vi "Interpolation Solver_worksheet.vi"(7 "method":T2(ring)=enum."Spline", 9 "factor":i32=11) -> ()   [LabVIEW 2021]
doc: "Demonstrates different types of interpolation on a set of raw data. The types of interpolation demonstrated in this example are Linear, Polynomial, Spline, and Rational."
uses:
  <vilib>/Analysis/NI_AALPro.lvlib
panel:
  out "Interpolated and sampled":string
  in  "Temp sampling":string="-2.2E-4\t4758.78\t1E-4\t2721.471\t-5E-5\t2008\t-5E-5\t1685\t1E-4\t1450\t1E-4\t1164.85\t-0.29989\t764.0274\n0.30011\t4462.235\t0.3\t2648\t0.30005\t1987.353\t0.30005\t1669\t1.1E-4\t1450\t0.29994\t1163\t-1.1E-4\t762.4022\n0.60005\t4148.875\t0.59999\t2535.23\t0.60005\t1930\t0.59994\t1632\t0.29994\t1442\t0.59999\t1154\t5E-5\t758.3495\n0.89999\t3924.31\t0.89999\t2443\t0.89993\t1879\t0.89999\t1596\t0.3\t1442\t0.9001\t1141\t0.29983\t759.8404\n1.19998\t3754.89\t1.19998\t2370\t1.19998\t1836\t1.19998\t1566\t0.59999\t1420\t1.20004\t1129.09\t0.3\t757.0791\n1.49993\t3615.25\t1.49993\t2311.24\t1.49998\t1800.059\t1.49998\t1539.437\t0.60005\t1419.15\t1.49993\t1118\t0.59994\t754.8484\n1.79992\t3502.73\t1.80003\t2261.312\t1.79987\t1771\t1.80003\t1516\t0.89999\t1395\t1.79992\t1108\t0.89999\t751.6615\n2.09992\t3405.49\t2.10003\t2219\t2.09992\t1747.25\t2.10036\t1496\t0.9001\t1395\t2.09992\t1099.24\t1.19998\t748.4732\n2.39997\t3317.85\t2.40008\t2181\t2.40008\t1728.235\t2.39997\t1478\t1.19988\t1373\t2.40002\t1092\t1.50004\t745.1494\n2.70008\t3247\t2.69997\t2147.36\t2.69997\t1712\t2.69991\t1460\t1.20004\t1373.353\t2.69997\t1085\t1.79998\t741.0916\n2.99991\t3177.43\t2.99996\t2122.941\t3.00007\t1699\t2.99996\t1447\t1.49998\t1354.235\t2.99991\t1079\t2.09997\t737.0983\n3.29996\t3122.62\t3.29996\t2096\t3.29996\t1687\t3.29996\t1435\t1.49998\t1354\t3.29996\t1073\t2.39992\t733.8118\n3.59995\t3072\t3.60001\t2074\t3.60001\t1676\t3.5999\t1425\t1.79992\t1338\t3.59995\t1068\t2.70002\t730.3677\n3.89995\t3024\t3.90011\t2054\t3.90001\t1666.537\t3.90006\t1416\t1.79998\t1336\t3.90011\t1063\t3.00007\t728.4455\n4.20006\t2982\t4.2\t2035.625\t4.19995\t1657.937\t4.2\t1406.937\t2.09986\t1319.059\t4.20006\t1059\t3.29996\t725.281\n4.49989\t2940.19\t4.49994\t2018.473\t4.49994\t1650\t4.49994\t1398\t2.09992\t1323\t4.49989\t1054.911\t3.60001\t723.3808\n4.79994\t2898\t4.79988\t2002.706\t4.79994\t1642.062\t4.80005\t1390.437\t2.39997\t1310\t4.79999\t1052\t3.90001\t721.5694\n5.09988\t2857.15\t5.09999\t1988\t5.10004\t1635\t5.09999\t1383.235\t2.40002\t1305\t5.09994\t1048.125\t4.2\t719.9192\n5.39993\t2811.62\t5.39999\t1974.187\t5.39999\t1629\t5.39999\t1377\t2.69997\t1298.57\t5.39999\t1046\t4.50005\t717.7494\n5.69998\t2746.67\t5.69998\t1962\t5.69998\t1622\t5.69993\t1371\t2.70002\t1291\t5.69998\t1043.84\t4.79994\t716.1806\n5.99998\t2712.765\t5.99987\t1950.04\t5.99998\t1616\t6.00009\t1364.789\t2.99996\t1278\t8.09995\t1018\t5.09994\t714.4917\n6.29997\t2692\t6.29987\t1939\t6.30003\t1610\t6.29992\t1359\t3.00002\t1287\t8.39989\t1015.588\t5.39999\t713.1643\n6.59997\t2672\t6.59992\t1928.157\t6.59986\t1604\t6.59992\t1354\t3.2999\t1265.792\t8.7\t1013\t5.70004\t711.2428\n6.89997\t2652.41\t6.90002\t1918\t6.89997\t1598\t6.89991\t1349\t3.30001\t1277.412\t9\t1011.39\t5.99998\t709.8922\n7.19996\t2632.31\t7.20002\t1908\t7.20007\t1592.78\t7.20007\t1344\t3.60001\t1269\t9.59993\t1007\t6.29992\t707.9154\n7.49996\t2613\t7.50001\t1899\t7.49991\t1587.19\t7.50001\t1339\t3.90001\t1260\t9.89998\t1004\t6.59992\t705.745\n7.79996\t2595.12\t7.79996\t1890\t7.79996\t1582\t7.80007\t1335\t4.19995\t1252\t10.19993\t1001\t6.89997\t704.6705\n8.09995\t2579\t8.09995\t1881\t8.10001\t1577\t8.0999\t1330\t4.49994\t1245\t10.49987\t998.8081\t7.19996\t702.9026\n8.39995\t2564\t8.40011\t1872\t8.39989\t1572.25\t8.39995\t1326\t4.79999\t1238\t10.80008\t996.05\t7.50001\t700.9308\n8.69994\t2549.75\t8.69989\t1865\t8.7\t1568\t8.70005\t1321\t5.09994\t1231\t11.09997\t994\t7.80001\t699.1752\n9\t2538\t8.99989\t1858\t9\t1563.882\t9\t1317.5\t5.39999\t1224\t11.39997\t992\t8.09995\t697.7639\n9.29994\t2527\t9.29994\t1852\t9.29994\t1559\t9.29994\t1313.706\t5.69993\t1217.294\t11.69991\t989.5833\t8.39989\t696.1505\n9.60004\t2516\t9.59993\t1845.634\t9.59999\t1555\t9.59993\t1310\t5.99998\t1211\t11.99996\t987.8235\t8.70005\t694.8553\n9.89987\t2508\t9.90004\t1840.48\t9.90004\t1551\t9.90009\t1306\t6.29997\t1205\t12.2999\t985.9565\t9\t692.7788\n10.19987\t2500.832\t10.19987\t1835.812\t10.19993\t1547.081\t10.19998\t1302\t6.60003\t1199.412\t12.59995\t983.7073\t9.29988\t691.7825\n10.50003\t2494.312\t10.49998\t1831\t10.49992\t1543.706\t10.50009\t1298.059\t6.89991\t1194\t12.89995\t981.303\t9.59993\t690.9664\n10.79997\t2489\t10.79992\t1826.059\t10.79986\t1539.824\t10.79997\t1295\t7.19996\t1188.812\t13.19989\t980\t9.90004\t689.5472\n11.10002\t2483\t11.09986\t1796.16\t11.09997\t1536\t11.10008\t1291\t7.50001\t1183\t13.50005\t977.6444\t10.19998\t688.6897\n11.40002\t2480.28\t11.39997\t1794.7\t11.39991\t1532\t11.39991\t1288\t7.7999\t1178\t13.79993\t974.67\t10.49998\t687.2567\n11.70002\t2475.706\t11.69996\t1790.53\t11.70002\t1529\t11.69991\t1284\t8.09995\t1172.294\t14.09999\t972\t10.79992\t686.3817\n11.99996\t2471\t12.00001\t1784.5\t11.9999\t1525\t12.00012\t1280\t8.4\t1167\t14.39998\t970\t11.09997\t684.9439\n12.2999\t2467\t12.29995\t1779.92\t12.29995\t1522\t12.29995\t1277\t8.7\t1161\t14.69998\t968\t11.40002\t683.9548\n12.60006\t2461.21\t12.6\t1775.3\t12.5999\t1518\t12.6\t1273.687\t8.99994\t1156\t14.99997\t965.81\t11.70007\t682.3112\n12.90006\t2456\t12.90006\t1770.63\t12.89995\t1514.86\t12.90006\t1270\t9.29999\t1152.494\t15.29997\t964\t11.99996\t681.3685\n13.19994\t2450\t13.2\t1765.062\t13.2\t1511\t13.19994\t1267\t9.59993\t1149\t15.60008\t961\t12.30012\t680.7712\n13.49983\t2444\t13.49994\t1761.42\t13.49994\t1508\t13.50005\t1263.36\t9.90004\t1146\t15.89991\t958.7826\t12.6\t679.2877\n13.8001\t2437\t13.79999\t1757.14\t13.79999\t1504.687\t13.79993\t1260\t10.19998\t1143\t16.1999\t957\t12.90016\t677.4835\n14.09988\t2429\t14.09993\t1756\t14.09999\t1501\t14.09993\t1257\t10.50003\t1140\t16.49996\t954.2941\t13.2\t676.5468\n14.39998\t2421.187\t14.39998\t1751.05\t14.39998\t1498\t14.40004\t1253.687\t10.80003\t1137\t16.80001\t952\t13.49999\t675.0764\n14.69998\t2414\t14.70003\t1746.097\t14.70003\t1495\t14.70003\t1250\t11.09991\t1134\t17.10006\t950\t13.80004\t674.3268\n14.99992\t2406\t14.99992\t1741.435\t14.99992\t1491.51\t14.99992\t1246.588\t11.39997\t1131.588\t17.39994\t947.8889\t14.10004\t672.6541\n15.30002\t2398\t15.30002\t1736.647\t15.29997\t1488.15\t15.30002\t1243\t11.69996\t1128.96\t17.4\t947\t14.39993\t671.7246\n15.60008\t2389\t15.59997\t1732\t15.60002\t1485.05\t15.60002\t1239\t11.99996\t1126\t17.69994\t945.7059\t14.69998\t670.1423\n15.89991\t2381\t15.89996\t1727.824\t15.89996\t1482\t15.89991\t1235.937\t12.30001\t1123.1\t17.69999\t945\t14.99997\t668.031\n16.19996\t2373.333\t16.20007\t1723\t16.1999\t1479\t16.19996\t1232\t12.59995\t1121\t17.99994\t943.55\t15.29997\t667.1016\n16.4999\t2365\t16.50001\t1718.687\t16.49996\t1475.875\t16.50006\t1227.55\t12.9\t1118\t17.99999\t944\t15.59997\t666.0608\n16.80006\t2357\t16.80001\t1714\t16.80001\t1472.529\t16.7999\t1224\t13.19994\t1115.62\t\t\t15.89985\t664.9405\n17.09989\t2348\t17.09995\t1709\t17.09995\t1469\t17.09989\t1220\t13.49994\t1113\t\t\t16.19996\t663.5747\n17.4\t2339\t17.39994\t1705\t17.39983\t1466\t17.39994\t1215.941\t13.80004\t1110\t\t\t16.50006\t662.5099\n17.69994\t2329.562\t17.69999\t1700\t17.69994\t1463\t17.69994\t1211.706\t14.09993\t1107\t\t\t16.79995\t661.2952\n17.99994\t2319.33\t17.99999\t1696\t17.99994\t1460\t17.99988\t1208\t14.39998\t1105\t\t\t17.10006\t660.3359\n\t\t\t\t\t\t\t\t14.69992\t1102\t\t\t17.40005\t658.4585\n\t\t\t\t\t\t\t\t14.99992\t1099.529\t\t\t17.7001\t657.2185\n\t\t\t\t\t\t\t\t15.29992\t1097\t\t\t18\t657.9\n\t\t\t\t\t\t\t\t15.60013\t1094\t\t\t\t\n\t\t\t\t\t\t\t\t15.89996\t1091\t\t\t\t\n\t\t\t\t\t\t\t\t16.1999\t1088.312\t\t\t\t\n\t\t\t\t\t\t\t\t16.50006\t1085\t\t\t\t\n\t\t\t\t\t\t\t\t16.80001\t1083\t\t\t\t\n\t\t\t\t\t\t\t\t17.1\t1080\t\t\t\t\n\t\t\t\t\t\t\t\t17.40011\t1077\t\t\t\t\n\t\t\t\t\t\t\t\t17.69994\t1074\t\t\t\t\n\t\t\t\t\t\t\t\t18\t1071.5"
  in  "Temp Resistance":string="-2.2E-4\t4758.78\t1E-4\t2721.471\t-5E-5\t2008\t-5E-5\t1685\t1E-4\t1450\t1E-4\t1164.85\t-0.29989\t764.0274\n0.30011\t4462.235\t0.3\t2648\t0.30005\t1987.353\t0.30005\t1669\t1.1E-4\t1450\t0.29994\t1163\t-1.1E-4\t762.4022\n0.60005\t4148.875\t0.59999\t2535.23\t0.60005\t1930\t0.59994\t1632\t0.29994\t1442\t0.59999\t1154\t5E-5\t758.3495\n0.89999\t3924.31\t0.89999\t2443\t0.89993\t1879\t0.89999\t1596\t0.3\t1442\t0.9001\t1141\t0.29983\t759.8404\n1.19998\t3754.89\t1.19998\t2370\t1.19998\t1836\t1.19998\t1566\t0.59999\t1420\t1.20004\t1129.09\t0.3\t757.0791\n1.49993\t3615.25\t1.49993\t2311.24\t1.49998\t1800.059\t1.49998\t1539.437\t0.60005\t1419.15\t1.49993\t1118\t0.59994\t754.8484\n1.79992\t3502.73\t1.80003\t2261.312\t1.79987\t1771\t1.80003\t1516\t0.89999\t1395\t1.79992\t1108\t0.89999\t751.6615\n2.09992\t3405.49\t2.10003\t2219\t2.09992\t1747.25\t2.10036\t1496\t0.9001\t1395\t2.09992\t1099.24\t1.19998\t748.4732\n2.39997\t3317.85\t2.40008\t2181\t2.40008\t1728.235\t2.39997\t1478\t1.19988\t1373\t2.40002\t1092\t1.50004\t745.1494\n2.70008\t3247\t2.69997\t2147.36\t2.69997\t1712\t2.69991\t1460\t1.20004\t1373.353\t2.69997\t1085\t1.79998\t741.0916\n2.99991\t3177.43\t2.99996\t2122.941\t3.00007\t1699\t2.99996\t1447\t1.49998\t1354.235\t2.99991\t1079\t2.09997\t737.0983\n3.29996\t3122.62\t3.29996\t2096\t3.29996\t1687\t3.29996\t1435\t1.49998\t1354\t3.29996\t1073\t2.39992\t733.8118\n3.59995\t3072\t3.60001\t2074\t3.60001\t1676\t3.5999\t1425\t1.79992\t1338\t3.59995\t1068\t2.70002\t730.3677\n3.89995\t3024\t3.90011\t2054\t3.90001\t1666.537\t3.90006\t1416\t1.79998\t1336\t3.90011\t1063\t3.00007\t728.4455\n4.20006\t2982\t4.2\t2035.625\t4.19995\t1657.937\t4.2\t1406.937\t2.09986\t1319.059\t4.20006\t1059\t3.29996\t725.281\n4.49989\t2940.19\t4.49994\t2018.473\t4.49994\t1650\t4.49994\t1398\t2.09992\t1323\t4.49989\t1054.911\t3.60001\t723.3808\n4.79994\t2898\t4.79988\t2002.706\t4.79994\t1642.062\t4.80005\t1390.437\t2.39997\t1310\t4.79999\t1052\t3.90001\t721.5694\n5.09988\t2857.15\t5.09999\t1988\t5.10004\t1635\t5.09999\t1383.235\t2.40002\t1305\t5.09994\t1048.125\t4.2\t719.9192\n5.39993\t2811.62\t5.39999\t1974.187\t5.39999\t1629\t5.39999\t1377\t2.69997\t1298.57\t5.39999\t1046\t4.50005\t717.7494\n5.69998\t2746.67\t5.69998\t1962\t5.69998\t1622\t5.69993\t1371\t2.70002\t1291\t5.69998\t1043.84\t4.79994\t716.1806\n5.99998\t2712.765\t5.99987\t1950.04\t5.99998\t1616\t6.00009\t1364.789\t2.99996\t1278\t8.09995\t1018\t5.09994\t714.4917\n6.29997\t2692\t6.29987\t1939\t6.30003\t1610\t6.29992\t1359\t3.00002\t1287\t8.39989\t1015.588\t5.39999\t713.1643\n6.59997\t2672\t6.59992\t1928.157\t6.59986\t1604\t6.59992\t1354\t3.2999\t1265.792\t8.7\t1013\t5.70004\t711.2428\n6.89997\t2652.41\t6.90002\t1918\t6.89997\t1598\t6.89991\t1349\t3.30001\t1277.412\t9\t1011.39\t5.99998\t709.8922\n7.19996\t2632.31\t7.20002\t1908\t7.20007\t1592.78\t7.20007\t1344\t3.60001\t1269\t9.59993\t1007\t6.29992\t707.9154\n7.49996\t2613\t7.50001\t1899\t7.49991\t1587.19\t7.50001\t1339\t3.90001\t1260\t9.89998\t1004\t6.59992\t705.745\n7.79996\t2595.12\t7.79996\t1890\t7.79996\t1582\t7.80007\t1335\t4.19995\t1252\t10.19993\t1001\t6.89997\t704.6705\n8.09995\t2579\t8.09995\t1881\t8.10001\t1577\t8.0999\t1330\t4.49994\t1245\t10.49987\t998.8081\t7.19996\t702.9026\n8.39995\t2564\t8.40011\t1872\t8.39989\t1572.25\t8.39995\t1326\t4.79999\t1238\t10.80008\t996.05\t7.50001\t700.9308\n8.69994\t2549.75\t8.69989\t1865\t8.7\t1568\t8.70005\t1321\t5.09994\t1231\t11.09997\t994\t7.80001\t699.1752\n9\t2538\t8.99989\t1858\t9\t1563.882\t9\t1317.5\t5.39999\t1224\t11.39997\t992\t8.09995\t697.7639\n9.29994\t2527\t9.29994\t1852\t9.29994\t1559\t9.29994\t1313.706\t5.69993\t1217.294\t11.69991\t989.5833\t8.39989\t696.1505\n9.60004\t2516\t9.59993\t1845.634\t9.59999\t1555\t9.59993\t1310\t5.99998\t1211\t11.99996\t987.8235\t8.70005\t694.8553\n9.89987\t2508\t9.90004\t1840.48\t9.90004\t1551\t9.90009\t1306\t6.29997\t1205\t12.2999\t985.9565\t9\t692.7788\n10.19987\t2500.832\t10.19987\t1835.812\t10.19993\t1547.081\t10.19998\t1302\t6.60003\t1199.412\t12.59995\t983.7073\t9.29988\t691.7825\n10.50003\t2494.312\t10.49998\t1831\t10.49992\t1543.706\t10.50009\t1298.059\t6.89991\t1194\t12.89995\t981.303\t9.59993\t690.9664\n10.79997\t2489\t10.79992\t1826.059\t10.79986\t1539.824\t10.79997\t1295\t7.19996\t1188.812\t13.19989\t980\t9.90004\t689.5472\n11.10002\t2483\t11.09986\t1796.16\t11.09997\t1536\t11.10008\t1291\t7.50001\t1183\t13.50005\t977.6444\t10.19998\t688.6897\n11.40002\t2480.28\t11.39997\t1794.7\t11.39991\t1532\t11.39991\t1288\t7.7999\t1178\t13.79993\t974.67\t10.49998\t687.2567\n11.70002\t2475.706\t11.69996\t1790.53\t11.70002\t1529\t11.69991\t1284\t8.09995\t1172.294\t14.09999\t972\t10.79992\t686.3817\n11.99996\t2471\t12.00001\t1784.5\t11.9999\t1525\t12.00012\t1280\t8.4\t1167\t14.39998\t970\t11.09997\t684.9439\n12.2999\t2467\t12.29995\t1779.92\t12.29995\t1522\t12.29995\t1277\t8.7\t1161\t14.69998\t968\t11.40002\t683.9548\n12.60006\t2461.21\t12.6\t1775.3\t12.5999\t1518\t12.6\t1273.687\t8.99994\t1156\t14.99997\t965.81\t11.70007\t682.3112\n12.90006\t2456\t12.90006\t1770.63\t12.89995\t1514.86\t12.90006\t1270\t9.29999\t1152.494\t15.29997\t964\t11.99996\t681.3685\n13.19994\t2450\t13.2\t1765.062\t13.2\t1511\t13.19994\t1267\t9.59993\t1149\t15.60008\t961\t12.30012\t680.7712\n13.49983\t2444\t13.49994\t1761.42\t13.49994\t1508\t13.50005\t1263.36\t9.90004\t1146\t15.89991\t958.7826\t12.6\t679.2877\n13.8001\t2437\t13.79999\t1757.14\t13.79999\t1504.687\t13.79993\t1260\t10.19998\t1143\t16.1999\t957\t12.90016\t677.4835\n14.09988\t2429\t14.09993\t1756\t14.09999\t1501\t14.09993\t1257\t10.50003\t1140\t16.49996\t954.2941\t13.2\t676.5468\n14.39998\t2421.187\t14.39998\t1751.05\t14.39998\t1498\t14.40004\t1253.687\t10.80003\t1137\t16.80001\t952\t13.49999\t675.0764\n14.69998\t2414\t14.70003\t1746.097\t14.70003\t1495\t14.70003\t1250\t11.09991\t1134\t17.10006\t950\t13.80004\t674.3268\n14.99992\t2406\t14.99992\t1741.435\t14.99992\t1491.51\t14.99992\t1246.588\t11.39997\t1131.588\t17.39994\t947.8889\t14.10004\t672.6541\n15.30002\t2398\t15.30002\t1736.647\t15.29997\t1488.15\t15.30002\t1243\t11.69996\t1128.96\t17.4\t947\t14.39993\t671.7246\n15.60008\t2389\t15.59997\t1732\t15.60002\t1485.05\t15.60002\t1239\t11.99996\t1126\t17.69994\t945.7059\t14.69998\t670.1423\n15.89991\t2381\t15.89996\t1727.824\t15.89996\t1482\t15.89991\t1235.937\t12.30001\t1123.1\t17.69999\t945\t14.99997\t668.031\n16.19996\t2373.333\t16.20007\t1723\t16.1999\t1479\t16.19996\t1232\t12.59995\t1121\t17.99994\t943.55\t15.29997\t667.1016\n16.4999\t2365\t16.50001\t1718.687\t16.49996\t1475.875\t16.50006\t1227.55\t12.9\t1118\t17.99999\t944\t15.59997\t666.0608\n16.80006\t2357\t16.80001\t1714\t16.80001\t1472.529\t16.7999\t1224\t13.19994\t1115.62\t\t\t15.89985\t664.9405\n17.09989\t2348\t17.09995\t1709\t17.09995\t1469\t17.09989\t1220\t13.49994\t1113\t\t\t16.19996\t663.5747\n17.4\t2339\t17.39994\t1705\t17.39983\t1466\t17.39994\t1215.941\t13.80004\t1110\t\t\t16.50006\t662.5099\n17.69994\t2329.562\t17.69999\t1700\t17.69994\t1463\t17.69994\t1211.706\t14.09993\t1107\t\t\t16.79995\t661.2952\n17.99994\t2319.33\t17.99999\t1696\t17.99994\t1460\t17.99988\t1208\t14.39998\t1105\t\t\t17.10006\t660.3359\n\t\t\t\t\t\t\t\t14.69992\t1102\t\t\t17.40005\t658.4585\n\t\t\t\t\t\t\t\t14.99992\t1099.529\t\t\t17.7001\t657.2185\n\t\t\t\t\t\t\t\t15.29992\t1097\t\t\t18\t657.9\n\t\t\t\t\t\t\t\t15.60013\t1094\t\t\t\t\n\t\t\t\t\t\t\t\t15.89996\t1091\t\t\t\t\n\t\t\t\t\t\t\t\t16.1999\t1088.312\t\t\t\t\n\t\t\t\t\t\t\t\t16.50006\t1085\t\t\t\t\n\t\t\t\t\t\t\t\t16.80001\t1083\t\t\t\t\n\t\t\t\t\t\t\t\t17.1\t1080\t\t\t\t\n\t\t\t\t\t\t\t\t17.40011\t1077\t\t\t\t\n\t\t\t\t\t\t\t\t17.69994\t1074\t\t\t\t\n\t\t\t\t\t\t\t\t18\t1071.5"
  out "error out":errorcluster
  out "Raw and Interpolated Data":T1(graph)=[{"Original Data (X,Y)"=[0.0, 1.2, 2.0, 3.0, 3.5, 4.0, 5.0], "Original Data (X,Y)"=[1.0, 2.700000047683716, 7.400000095367432, 150.0, 140.0, 80.0, 220.0]}, {"Original Data (X,Y)"=[0.0, 0.09999999999999999, 0.19999999999999998, 0.3, 0.39999999999999997, 0.5, 0.6, 0.7000000000000001, 0.7999999999999999, 0.8999999999999999, 1.0, 1.0999999999999999, 1.2, 1.2666666666666666, 1.3333333333333333, 1.4, 1.4666666666666666, 1.5333333333333334, 1.6, 1.6666666666666665, 1.7333333333333334, 1.8, 1.8666666666666667, 1.9333333333333333, 2.0, 2.0833333333333335, 2.1666666666666665, 2.25, 2.3333333333333335, 2.4166666666666665, 2.5, 2.5833333333333335, 2.6666666666666665, 2.75, 2.8333333333333335, 2.9166666666666665, 3.0, 3.041666666666667, 3.083333333333333, 3.125, 3.166666666666667, 3.208333333333333, 3.25, 3.291666666666667, 3.333333333333333, 3.375, 3.416666666666667, 3.458333333333333, 3.5, 3.5416666666666665, 3.5833333333333335, 3.625, 3.6666666666666665, 3.7083333333333335, 3.75, 3.7916666666666665, 3.8333333333333335, 3.875, 3.9166666666666665, 3.9583333333333335, 4.0, 4.083333333333333, 4.166666666666667, 4.25, 4.333333333333333, 4.416666666666667, 4.5, 4.583333333333333, 4.666666666666667, 4.75, 4.833333333333333, 4.916666666666667, 5.0], "Original Data (X,Y)"=[1.0, 2.3924029604023143, 3.732327475080349, 4.967295098309824, 6.044827384366458, 6.912445887525974, 7.5176721620640885, 7.8080277622565255, 7.7310342423790015, 7.23421315670724, 6.265086059516957, 4.771174505083877, 2.700000047683716, 1.000579506543195, -0.82639929721429, -2.628609582342879, -4.253724567596707, -5.549417471729917, -6.363361513496636, -6.54322991165102, -5.936695884947188, -4.3914326521392875, -1.755113431981461, 2.124588556772159, 7.400000095367432, 16.068903365453245, 26.733298416919904, 38.96987026382418, 52.35530392022265, 66.46628440017192, 80.87949671772876, 95.17162588694978, 108.91935692189152, 121.69937483661082, 133.08836464516423, 142.66301136160837, 150.0, 152.7067362173637, 154.75321245875486, 156.1444120142, 156.8853181737255, 156.9809142273579, 156.43618346512363, 155.25610917704915, 153.44567465316098, 151.0098631834855, 147.95365805804917, 144.28204256687857, 140.0, 135.13403211106163, 129.7967145081979, 124.12214126316489, 118.24440644771866, 112.2976041336152, 106.41582839261069, 100.73317329646115, 95.38373291692258, 90.50160132575115, 86.22087259470287, 82.67564079553378, 80.0, 77.5593153292216, 78.79880926821149, 83.38392012517251, 90.98008620830757, 101.25274582581966, 113.86733728591145, 128.48929889678593, 144.78406896664615, 162.41708580369465, 181.0537877161345, 200.3596130121688, 220.0]}]
  # "Example\n1. Paste raw data table of Temperature Resistance in the first window.\n2. Paste sampling temperatures in the second window.\n3. Run the program;\n      i) the interpolation of the raw data is performed\n      ii) the interpolation of the sampled number is performed\n4. The third window will show a table of interpolated Sampled T and corresponding R\n\nNote: \n(1) This program can be used to create a thermometer calibration file from a raw data.\n(2) For RTD like Cernox, RuO2, an alternative method, probably better, with Cheby fitting is available."
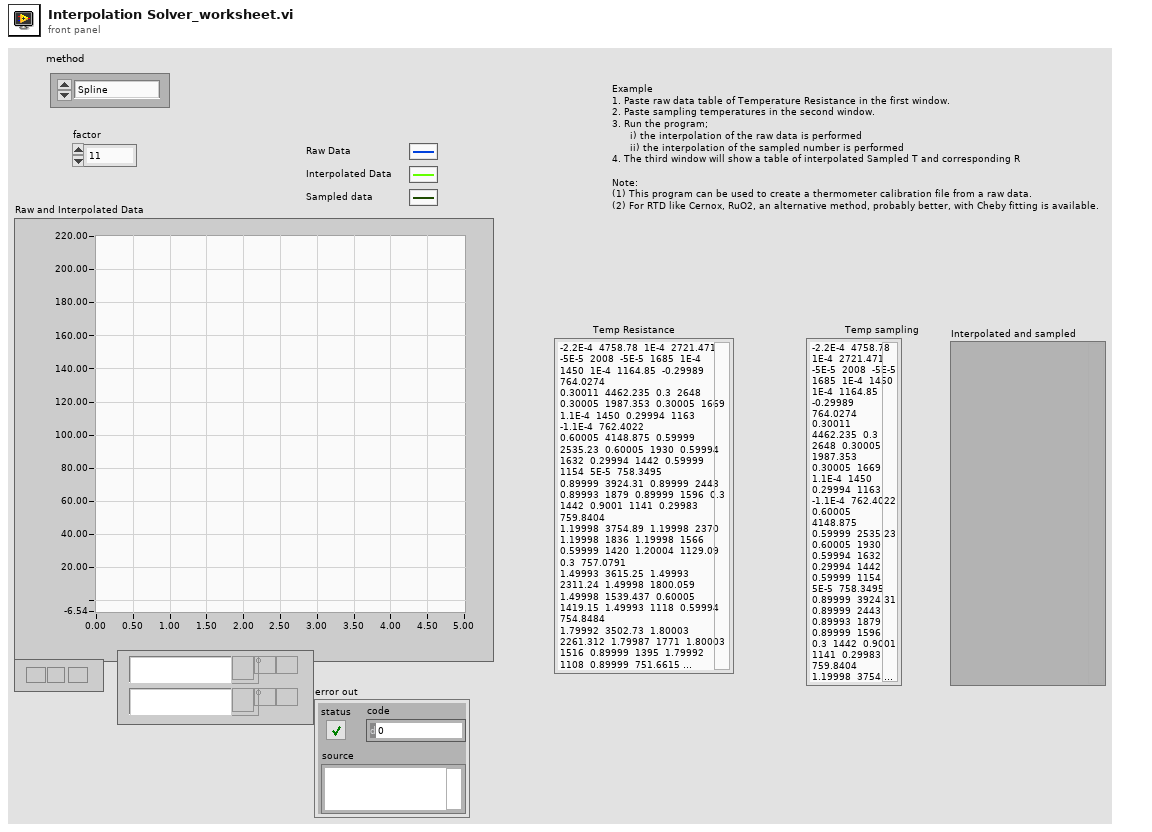
[diagram p1: front panel]
types:
  T1 = cluster{"Original Data (X,Y)":dbl[], "Original Data (X,Y)":dbl[]}[]
  T2 = enum16{"Linear", "Polynomial", "Spline", "Rational"}
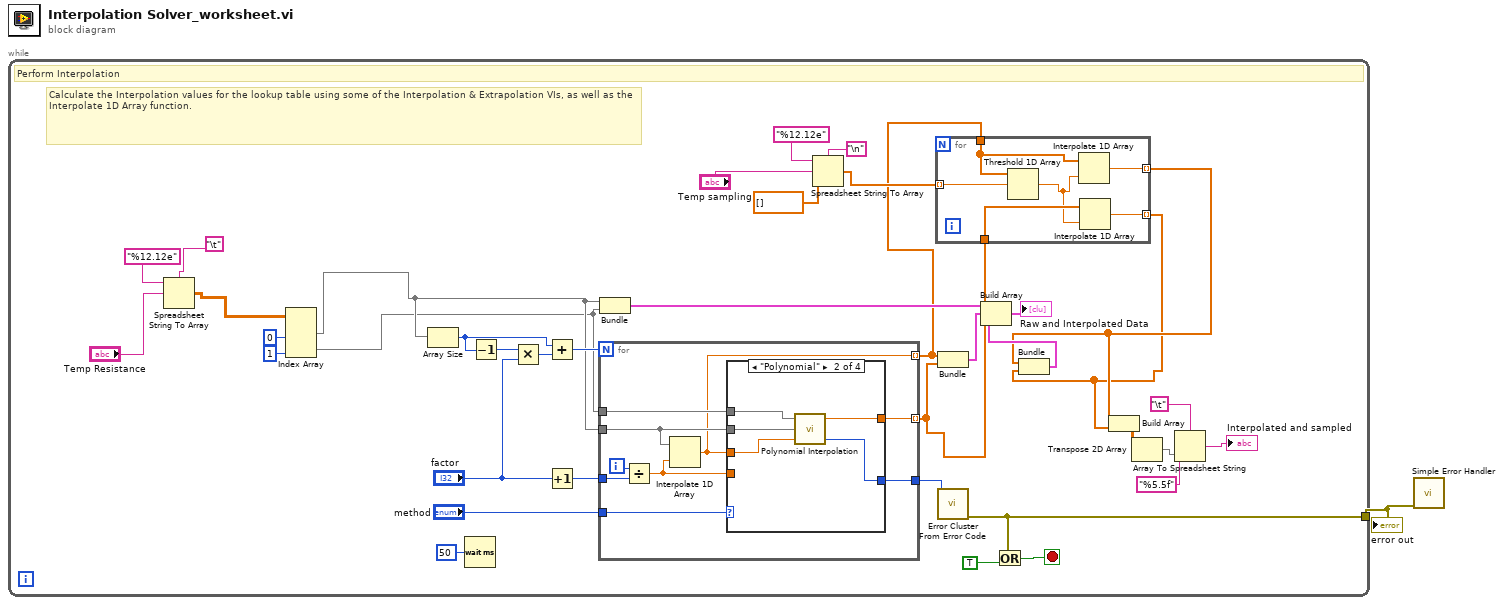
[diagram p0: block diagram]
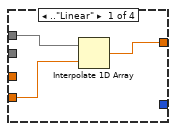
[diagram p2: hidden frame]
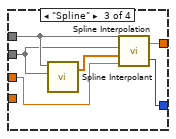
[diagram p3: hidden frame]
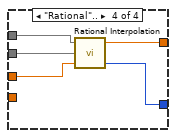
[diagram p4: hidden frame]
diagram:
  n1 = while {
    tunnel: [w26] -> w1
    stop <- w27 stop-if-true
    # "Calculate the Interpolation values for the lookup table using some of the Interpolation & Extrapolation VIs, as well as the Interpolate 1D Array function."
    # "Perform Interpolation"
    n2 = Spreadsheet String To Array(delimiter (Tab)="\t", format string="%12.12e", spreadsheet string="Temp Resistance") -> (array=w21:dbl[][])  [unwired: 1 in]
    n3 = Index Array(array=w21, index (col) #1=0 ("disabled index (col)"), index (col) #2=1 ("index (col)")) -> (element #1=w18:dbl[], element #2=w17:dbl[])  [unwired: 2 in]
    n4 = Array Size(array=w18) -> (size(s)=w31:i32)
    n5 = Wait (ms)(milliseconds to wait=u32 50) -> ()  [unwired: 1 out]
    n6 = Decrement(x=w31) -> (x-1=w34:i32)
    n7 = Multiply(x=w34, y="factor") -> (x*y=w32:i32)
    n8 = Add(x=w31, y=w32) -> (x+y=w30:i32)
    n9 = Increment(x="factor") -> (x+1=w33:i32)
    n10 = for {
      N: w30 -> [_]
      tunnel: w17 -> [w54]
      tunnel: w18 -> [w48]
      tunnel: [w53] -> w28
      tunnel: "method" -> [w49]
      tunnel: w33 -> [w51]
      tunnel: [w50] -> w10 mode=indexing
      tunnel: [w47] -> w11 mode=indexing
      i -> [w52]
      n11 = Divide(x=w52, y=w51) -> (x/y=w46:dbl)
      n12 = Interpolate 1D Array(1:w46, 2:w48) -> (0:w47:dbl)
      n13 = case shown="\"Polynomial\"" w49 {
        tunnel: w47 -> [_ w62 w65 w69]
        tunnel: [w56 w61 w63 w71] -> w50
        tunnel: [_ w60 w64 w70] -> w53
        tunnel: w48 -> [_ w59 w66 w72]
        tunnel: w54 -> [w57 w58 w68 w73]
        tunnel: w46 -> [w55 _ _ _]
        frame .."Linear" {
          n14 = Interpolate 1D Array(1:w55, 2:w57) -> (0:w56:dbl)
        }
        frame "Polynomial" {
          n15 = call <vilib>:"Polynomial Interpolation.vi"("x value"=w62, "X"=w59, "Y"=w58) -> ("error"=w60:i32, "interpolation value"=w61:dbl)  [unwired: 1 out]
        }
        frame "Spline" {
          n16 = call <vilib>:"Spline Interpolant.vi"("X"=w66, "Y"=w68) -> ("Interpolant"=w67:dbl[])  [unwired: 2 in, 1 out]
          n17 = call <vilib>:"Spline Interpolation.vi"("x value"=w65, "Interpolant"=w67, "X"=w66, "Y"=w68) -> ("error"=w64:i32, "interpolation value"=w63:dbl)
        }
        frame "Rational".. {
          n18 = call <vilib>:"Rational Interpolation.vi"("x value"=w69, "X"=w72, "Y"=w73) -> ("error"=w70:i32, "interpolation value"=w71:dbl)  [unwired: 1 out]
        }
      }
    }
    n19 = Bundle(w18, w17) -> (w35:cluster{dbl[], dbl[]})  [unwired: 1 in]
    n20 = Spreadsheet String To Array(delimiter (Tab)="\n", format string="%12.12e", spreadsheet string="Temp sampling", array type (2D Dbl)=dbl[] []) -> (array=w12:dbl[])
    n21 = for {
      tunnel: w12 -> [w45] mode=indexing
      tunnel: w11 -> [w44]
      tunnel: w10 -> [w43]
      tunnel: [w41] -> w8 mode=indexing
      tunnel: [w40] -> w7 mode=indexing
      n22 = Threshold 1D Array(2:w45, 3:w44) -> (0:w42:dbl)  [unwired: 1 in]
      n23 = Interpolate 1D Array(1:w42, 2:w44) -> (0:w41:dbl)
      n24 = Interpolate 1D Array(1:w42, 2:w43) -> (0:w40:dbl)
    }
    n25 = Bundle(w11, w10) -> (w36:cluster{dbl[], dbl[]})  [unwired: 1 in]
    n26 = call <vilib>:"Error Cluster From Error Code.vi"("error code (0)"=w28) -> ("error out"=w26:errorcluster)  [unwired: 8 in]
    n27 = Or(x=w26, y=TRUE) -> (x .or. y?=w27:bool)
    n28 = Bundle(w8, w7) -> (w9:cluster{dbl[], dbl[]})  [unwired: 1 in]
    n29 = Build Array(w35, w36, w9) -> (→"Raw and Interpolated Data":cluster{dbl[], dbl[]}[])
    n30 = Build Array(w8, w7) -> (w5:dbl[][])
    n31 = Transpose 2D Array(2D array=w5) -> (transposed array=w6:dbl[][])
    n32 = Array To Spreadsheet String(delimiter (Tab)="\t", array=w6, 3:"%5.5f" ("format string")) -> (spreadsheet string=→"Interpolated and sampled":string)
  }
  "error out" <- w1
  n33 = call <vilib>:"Simple Error Handler.vi"("error in (no error)"=w1) -> ()  [unwired: 4 in, 5 out]
